vi "Go-Home.vi"() -> ()   [LabVIEW 2019]
panel:
  out "回起始點?":bool
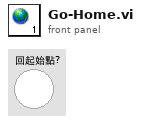
[diagram p1: front panel]
diagram:
